vi "String Included.vi"() -> (0 "error out":errorcluster)   [LabVIEW 2017, in "Assertion.Tests.lvlib" / "Assert String Contains String.lvlib"]
uses:
  Assert String Contains String.lvlib
  Assertion/Assertion.lvlib
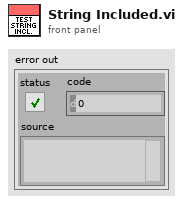
[diagram p1: front panel]
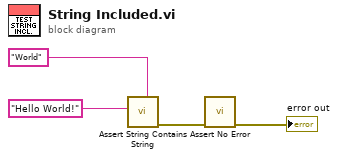
[diagram p0: block diagram]
diagram:
  n1 = call "Assert String Contains String.vi"("Needle"="World", "Haystack"="Hello World!") -> ("error out"=w2:errorcluster)  [unwired: 9 in]
  n2 = call "Assert No Error.vi"("error in (no error)"=w2) -> ("error out"=→"error out":errorcluster)  [unwired: 10 in]
